vi "AdventofCodeDay3.vi"() -> ()   [LabVIEW 2019]
panel:
  out "Solution 1":i32
  in  "String":string
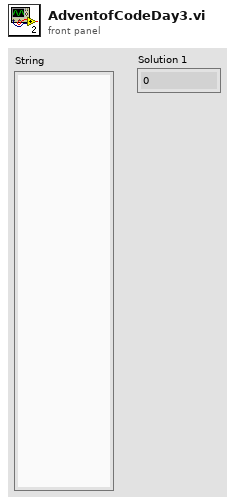
[diagram p1: front panel]
types:
  T1 = enum16{"Native", "Native Command Line", "UNIX", "Macintosh", "DOS"}
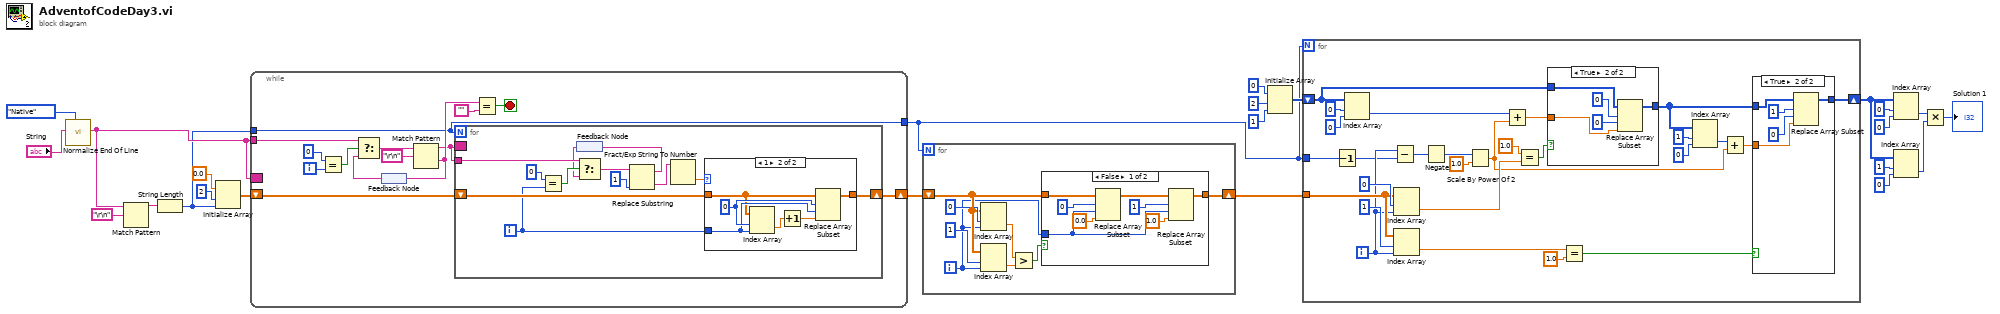
[diagram p0: block diagram]
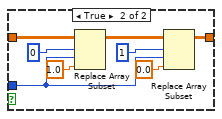
[diagram p4: hidden frame]
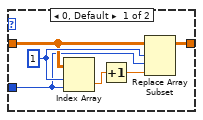
[diagram p5: hidden frame]
diagram:
  n1 = call <vilib>:"Normalize End Of Line.vi"("end of line (Native)"=T1."Native", "string in"="String") -> ("string out"=w4:string)  [unwired: 6 in]
  n2 = Match Pattern(string=w4, regular expression="\r\n") -> (before substring=w3:string)  [unwired: 1 in, 3 out]
  n3 = String Length(string=w3) -> (length=w2:i32)
  n4 = Initialize Array(0.0 ("element"), 2 ("dimension size"), w2) -> (w20:dbl[][])
  n5 = while {
    tunnel: w4 -> [w31]
    shift-right: [w37] -> w19
    shift-left: w20 -> [w38]
    border: w4 -> [_]
    tunnel: w2 -> [w25]
    tunnel: [w25] -> w1
    i -> [w34]
    stop <- w36 stop-if-true
    n6 = Equal?(x=0, y=w34) -> (x = y?=w32:bool)
    n7 = feedback #1() -> (w28:string)
    n8 = Select(t=w31, s=w32, f=w28) -> (s? t:f=w29:string)
    n9 = Match Pattern(string=w29, regular expression="\r\n") -> (before substring=w26:string, after substring=w27:string)  [unwired: 1 in, 2 out]
    n10 = feedback-in #1(w27) -> ()
    n11 = for {
      N: w25 -> [_]
      tunnel: w26 -> [w41]
      shift-right: [w47] -> w37
      shift-left: w38 -> [w46]
      border: w26 -> [_]
      i -> [w44]
      n12 = Equal?(x=0, y=w44) -> (x = y?=w45:bool)
      n13 = feedback #2() -> (w39:string)
      n14 = Select(t=w41, s=w45, f=w39) -> (s? t:f=w42:string)
      n15 = Replace Substring(2:1 ("length (len. of substring)"), 5:w42) -> (0:w48:string, 1:w40:string)  [unwired: 2 in]
      n16 = feedback-in #2(w40) -> ()
      n17 = Fract/Exp String To Number(string=w48) -> (number=w49:dbl)  [unwired: 3 in, 1 out]
      n18 = case shown="1" w49 {
        tunnel: [w52 w59] -> w47
        tunnel: w46 -> [w53 w57]
        tunnel: w44 -> [w51 w58]
        frame 0, Default {
          w55 = 1 ("index (row)")
          n19 = Index Array(array=w53, index (row)=w55, index (col)=w51) -> (element=w56:dbl)
          n20 = Increment(x=w56) -> (x+1=w54:dbl)
          n21 = Replace Array Subset(array=w53, new element=w54, index (row)=w55, index (col)=w51) -> (w52:dbl[][])
        }
        frame 1 {
          w61 = 0 ("index (row)")
          n22 = Index Array(array=w57, index (row)=w61, index (col)=w58) -> (element=w62:dbl)
          n23 = Increment(x=w62) -> (x+1=w60:dbl)
          n24 = Replace Array Subset(array=w57, new element=w60, index (row)=w61, index (col)=w58) -> (w59:dbl[][])
        }
      }
    }
    n25 = Equal?(x=w27, y="") -> (x = y?=w36:bool)
  }
  n26 = for {
    N: w1 -> [_]
    shift-right: [w63] -> w6
    shift-left: w19 -> [w65]
    i -> [w64]
    n27 = Index Array(array=w65, index (row)=0 ("index"), index (col)=w64) -> (element=w70:dbl)
    n28 = Index Array(array=w65, index (row)=1 ("index"), index (col)=w64) -> (element=w69:dbl)
    n29 = Greater?(x=w70, y=w69) -> (0:w66:bool)
    n30 = case shown="False" w66 {
      tunnel: w65 -> [w77 w86]
      tunnel: w64 -> [w73 w79]
      tunnel: [w74 w80] -> w63
      frame False {
        n31 = Replace Array Subset(array=w77, new element=0.0 ("new element/subarray"), index (row)=0 ("disabled index (row)"), index (col)=w73) -> (w75:dbl[][])
        n32 = Replace Array Subset(array=w75, new element=1.0 ("new element/subarray"), index (row)=1 ("disabled index (row)"), index (col)=w73) -> (w74:dbl[][])
      }
      frame True {
        n33 = Replace Array Subset(array=w86, new element=1.0 ("new element/subarray"), index (row)=0 ("disabled index (row)"), index (col)=w79) -> (w81:dbl[][])
        n34 = Replace Array Subset(array=w81, new element=0.0 ("new element/subarray"), index (row)=1 ("disabled index (row)"), index (col)=w79) -> (w80:dbl[][])
      }
    }
  }
  n35 = Initialize Array(0 ("element"), 2 ("dimension size"), 1 ("dimension size")) -> (w15:i32[][])
  n36 = for {
    N: w1 -> [_]
    shift-right: [w89] -> w13
    shift-left: w15 -> [w91]
    tunnel: w6 -> [w111]
    tunnel: w1 -> [w87]
    i -> [w103]
    n37 = Decrement(x=w87) -> (x-1=w88:i32)
    n38 = Index Array(array=w91, index (row)=0, index (col)=0 ("disabled index (col)")) -> (element=w104:i32)
    n39 = Subtract(x=w103, y=w88) -> (x-y=w102:i32)
    n40 = Index Array(array=w111, index (row)=0 ("index"), index (col)=w103) -> (element=w110:dbl)
    n41 = Index Array(array=w111, index (row)=1 ("index"), index (col)=w103) -> (element=w100:dbl)
    n42 = Negate(x=w102) -> (-x=w101:i32)
    n43 = Scale By Power Of 2(n=w101, x=1.0) -> (x*2^n=w94:dbl)
    n44 = Add(x=w104, y=w94) -> (x+y=w97:dbl)
    n45 = Equal?(x=1.0, y=w110) -> (x = y?=w108:bool)
    n46 = case shown="True" w108 {
      tunnel: w91 -> [w120 w125]
      tunnel: [w120 w124] -> w90
      tunnel: w97 -> [_ w121]
      frame False {
      }
      frame True {
        n47 = Replace Array Subset(array=w125, new element=w121, index (row)=0, index (col)=0) -> (w124:i32[][])
      }
    }
    n48 = Equal?(x=w100, y=1.0) -> (x = y?=w99:bool)
    n49 = Index Array(array=w90, index (row)=1, index (col)=0 ("disabled index (col)")) -> (element=w93:i32)
    n50 = Add(x=w93, y=w94) -> (x+y=w92:dbl)
    n51 = case shown="True" w99 {
      tunnel: w90 -> [w114 w119]
      tunnel: [w114 w118] -> w89
      tunnel: w92 -> [_ w115]
      frame False {
      }
      frame True {
        n52 = Replace Array Subset(array=w119, new element=w115, index (row)=1, index (col)=0) -> (w118:i32[][])
      }
    }
  }
  n53 = Index Array(array=w13, index (row)=0, index (col)=0 ("disabled index (col)")) -> (element=w8:i32)
  n54 = Index Array(array=w13, index (row)=1, index (col)=0 ("disabled index (col)")) -> (element=w14:i32)
  n55 = Multiply(x=w8, y=w14) -> (x*y=→"Solution 1":i32)
